vi "2_For_loop.vi"() -> ()   [LabVIEW 2019]
panel:
  out "Tablica z całkowitymi (I8)\nliczbami przypadkowymi \nw zakresie od 0 do 100.":i8[][](array[numeric])
  in  "Wymiar y":i8=2 min=1 max=10 step=1
  in  "Wymiar x":i8=2 min=1 max=10 step=1
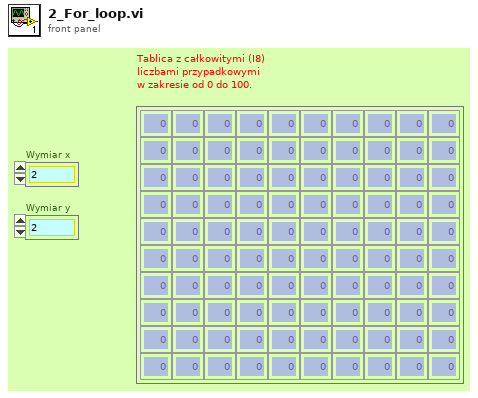
[diagram p1: front panel]
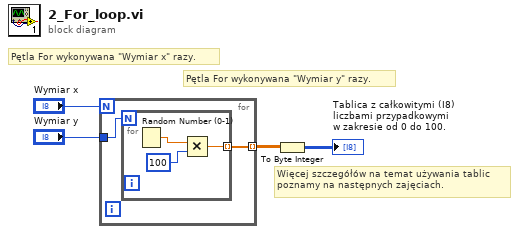
[diagram p0: block diagram]
diagram:
  # "Więcej szczegółów na temat używania tablic\npoznamy na następnych zajęciach."
  # "Pętla For wykonywana \"Wymiar y\" razy."
  # "Pętla For wykonywana \"Wymiar x\" razy."
  n1 = for {
    N: "Wymiar x" -> [_]
    tunnel: "Wymiar y" -> [w6]
    tunnel: [w5] -> w2 mode=indexing
    n2 = for {
      N: w6 -> [_]
      tunnel: [w7] -> w5 mode=indexing
      n3 = Random Number (0-1)() -> (number: 0 to 1=w9:dbl)
      n4 = Multiply(x=w9, y=i8 100) -> (x*y=w7:dbl)
    }
  }
  n5 = To Byte Integer(number=w2) -> (8bit integer=→"Tablica z całkowitymi (I8)\nliczbami przypadkowymi \nw zakresie od 0 do 100.":i8[][])
